vi "Write Interactive.vi"(8 "error in (no error)":errorcluster, 10 "Interactive":bool, 11 "DefineSuite in":refnum<class "DestroySuite.lvclass">) -> (0 "error out":errorcluster, 3 "DefineSuite out":refnum<class "DestroySuite.lvclass">)   [LabVIEW 2021]
uses:
  DestroySuite.lvclass/DestroySuite.ctl
  DestroySuite.lvclass
  C:/Repositories/LVOS/Bananas/lv-src/Bananas/DestroySuite/DestroySuite.lvclass
  C:/Repositories/LVOS/Bananas/lv-src/Bananas/BananaPeel/BananaPeel.lvclass
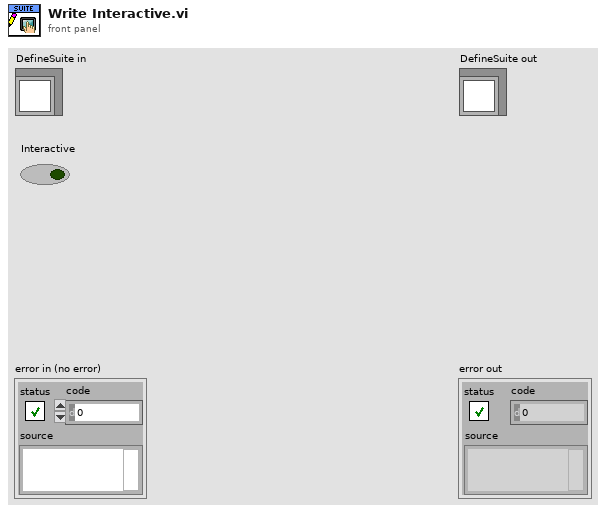
[diagram p1: front panel]
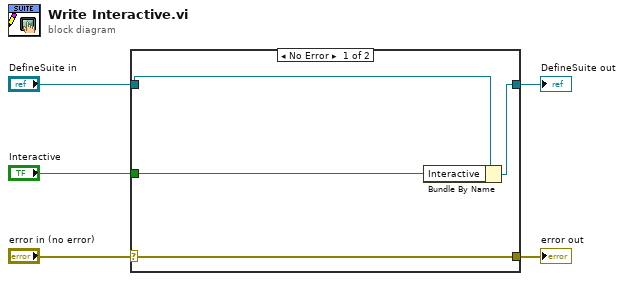
[diagram p0: block diagram]
diagram:
  n1 = case shown="No Error" "error in (no error)" {
    selector: "error in (no error)" -> [w9 w10]
    tunnel: [w9 w10] -> w4
    tunnel: [w7 w11] -> w2
    tunnel: "DefineSuite in" -> [w8 w11]
    tunnel: "Interactive" -> [w6 _]
    frame No Error {
      n2 = Bundle By Name(cluster=w8, "Interactive"=w6) -> (w7:refnum<class "DestroySuite.lvclass">)
    }
    frame Error {
    }
  }
  "error out" <- w4
  "DefineSuite out" <- w2
